vi "SubVI Make MT waveform.vi"(0 "t0":dbl, 1 "dt":dbl=1.0, 2 "Y":cdb[](array[numeric])) -> (3 "输出MT波形":cluster{"t0":dbl, "dt":dbl, "Y":cdb[]})   [LabVIEW 2015]
panel:
  # "Use this VI to make a waveform cluster that is suitable for Modulation Toolkit VIs."
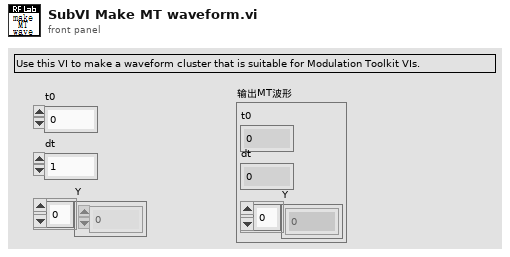
[diagram p1: front panel]
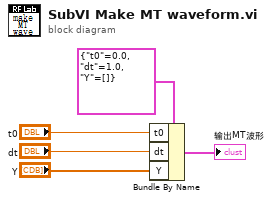
[diagram p0: block diagram]
diagram:
  n1 = Bundle By Name(cluster=cluster{"t0":dbl, "dt":dbl, "Y":cdb[]} {"t0"=0.0, "dt"=1.0, "Y"=[]} ("IQ data (complex) in"), "t0"="t0", "dt"="dt", "Y"="Y") -> (→"输出MT波形":cluster{"t0":dbl, "dt":dbl, "Y":cdb[]})
